vi "FringeTrackerAlignRaster.vi"(4 "goToPeak":i32(ring) items=["No", "Yes"], 6 "channel":i32(ring) items=["WL", "SPEC"], 8 "error in (no error)":errorcluster, 11 "FringeTracker Name":string="TipTiltMirror[1]") -> (0 "error out":errorcluster caption="error in (no error)", 3 "FringeTracker Name out":string, 5 "yOffset":dbl, 7 "xOffset":dbl)   [LabVIEW 2009]
uses:
  lib/lvrtc.dll
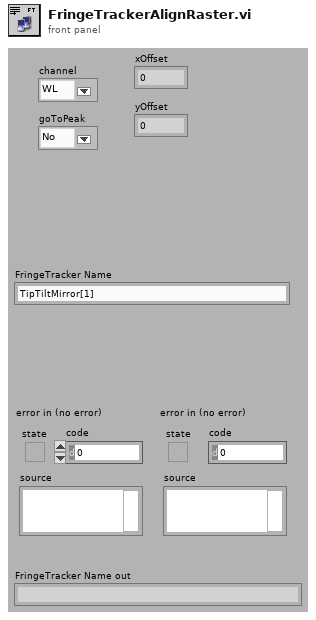
[diagram p1: front panel]
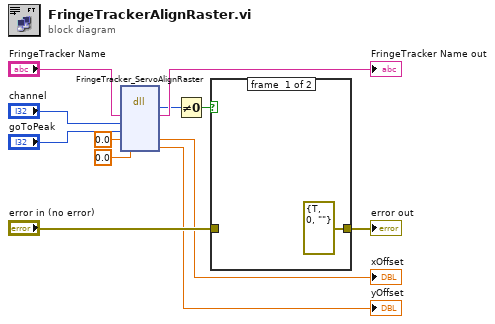
[diagram p0: block diagram]
diagram:
  n1 = dll-call lib="C:/Ohana/LV2009/OhanaOS-LV81/Instruments/RTC/Api/lib/lvrtc.dll" fn="FringeTracker_ServoAlignRaster"("FringeTrackerName"="FringeTracker Name", "channel"="channel", "goToPeak"="goToPeak", "xOffset"=0.0, "yOffset"=0.0) -> ("return type"=w9:i32, "FringeTrackerName"=→"FringeTracker Name out":string, "xOffset"=→"xOffset":dbl, "yOffset"=→"yOffset":dbl)  [unwired: 5 in, 2 out]
  n2 = Not Equal To 0?(x=w9) -> (x != 0?=w8:bool)
  n3 = case shown="False" w8 {
    tunnel: "error in (no error)" -> [_ w14]
    tunnel: [errorcluster {"status"=TRUE, "code"=0, "source"=""} ("error in (no error)") w14] -> w7
    frame #0 {
    }
    frame #1 {
    }
  }
  "error out" <- w7
